vi "OAT Get Slow Roll Vectors.vi"   [LabVIEW 2017]
doc: "computes the vector references of the specified orders from the slow roll vibration signals. The vector references are used for displacement transducer signals to compensate shaft bow or runout. You can use this polymorphic VI to get references from a single channel or from N channels. The data type you wire to the <B>scaled signal [EU]</B> input determines the polymorphic instance to use."
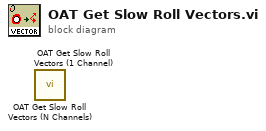
[diagram p0: block diagram]
diagram:
  n1 = call <vilib>:"OAT Get Slow Roll Vectors (N Channels).vi"() -> ()  [unwired: 14 in, 2 out]
  n2 = call <vilib>:"OAT Get Slow Roll Vectors (1 Channel).vi"() -> ()  [unwired: 14 in, 2 out]
